vi "Update Controller State.vi"(8 "error in (no error)":errorcluster, 11 "Car Wash Controller Actor in":refnum<class "Car Wash Controller Actor.lvclass">) -> (0 "error out":errorcluster, 3 "Car Wash Controller Actor out":refnum<class "Car Wash Controller Actor.lvclass">)   [LabVIEW 2019, in "Car Wash Controller Actor.lvlib" / "Car Wash Controller Actor.lvclass"]
uses:
  Car Wash Controller Actor.lvclass
  C:/Program Files (x86)/National Instruments/LabVIEW 2019/vi.lib/ActorFramework/Actor/Actor.lvclass
  <vilib>/ActorFramework/Actor/Actor.lvclass/Actor.ctl
  <vilib>/ActorFramework/Message Enqueuer/Message Enqueuer.lvclass/Message Enqueuer.ctl
  Car Wash Controller Actor.lvclass/Car Wash Controller Actor.ctl
  Sim Entry Console Actor/Sim Entry Console Actor/Wash steps selection -Buttons.ctl
  Configuration Database Actor/Configuration Database Actor/DB type.ctl
  Configuration Database Actor/Configuration Database Actor Messages/Select DB Msg/Select DB Msg.lvclass/Select DB Msg.ctl
  Vehicle Position Simulation/Vehicle Position Simulation Messages/Update Vehicle Position Simulation Msg/Update Vehicle Position Simulation Msg.lvclass/Update Vehicle Position Simulation Msg.ctl
  Simulated Wash Display Console Actor/Simulated Wash Display Console Actor Messages/Update Wash Entry Msg/Update Wash Entry Msg.lvclass/Update Wash Entry Msg.ctl
  Simulated Wash Display Console Actor/Simulated Wash Display Console Actor Messages/Update Vehicle Out of Position Msg/Update Vehicle Out of Position Msg.lvclass/Update Vehicle Out of Position Msg.ctl
  Simulated Wash Display Console Actor/Simulated Wash Display Console Actor Messages/Update Car Wash Indicators Msg/Update Car Wash Indicators Msg.lvclass/Update Car Wash Indicators Msg.ctl
  Simulated Wash Display Console Actor/Simulated Wash Display Console Actor Messages/Update Time Remaining Msg/Update Time Remaining Msg.lvclass/Update Time Remaining Msg.ctl
  Sim Entry Console Actor/Simulated Entry Console Actor Messages/Enable Start Msg/Enable Start Msg.lvclass/Enable Start Msg.ctl
  Sim Entry Console Actor/Simulated Entry Console Actor Messages/Enable Wash steps Msg/Enable Wash steps Msg.lvclass/Enable Wash steps Msg.ctl
  State -Enum.ctl
  Car Wash Controller Actor Messages/Set State Msg/Set State Msg.lvclass/Set State Msg.ctl
  <vilib>/ActorFramework/Message Enqueuer/Init from Existing Queue.vi
  <vilib>/ActorFramework/Message Enqueuer/Enqueue.vi
  Configuration Database Actor/Configuration Database Actor Messages/Select DB Msg/Select DB Msg.lvclass
  C:/Program Files (x86)/National Instruments/LabVIEW 2019/vi.lib/ActorFramework/Message/Message.lvclass
  Vehicle Position Simulation/Vehicle Position Simulation Messages/Update Vehicle Position Simulation Msg/Update Vehicle Position Simulation Msg.lvclass
  Simulated Wash Display Console Actor/Simulated Wash Display Console Actor Messages/Update Wash Entry Msg/Update Wash Entry Msg.lvclass
  Simulated Wash Display Console Actor/Simulated Wash Display Console Actor Messages/Update Vehicle Out of Position Msg/Update Vehicle Out of Position Msg.lvclass
  Simulated Wash Display Console Actor/Simulated Wash Display Console Actor Messages/Update Car Wash Indicators Msg/Update Car Wash Indicators Msg.lvclass
  Simulated Wash Display Console Actor/Simulated Wash Display Console Actor Messages/Update Time Remaining Msg/Update Time Remaining Msg.lvclass
  Sim Entry Console Actor/Simulated Entry Console Actor Messages/Enable Start Msg/Enable Start Msg.lvclass
  Sim Entry Console Actor/Simulated Entry Console Actor Messages/Enable Wash steps Msg/Enable Wash steps Msg.lvclass
  Configuration Database Actor/Configuration Database Actor Messages/Read Record Msg/Read Record Msg.lvclass
  Vehicle Position Simulation/Vehicle Position Simulation Messages/Check Vehicle Exit Msg/Check Vehicle Exit Msg.lvclass
  Car Wash Controller Actor Messages/Set State Msg/Set State Msg.lvclass
  <vilib>/ActorFramework/Message Priority Queue/Priority Enqueue.vi
  <vilib>/ActorFramework/Message Enqueuer/Message Enqueuer.lvclass
  <vilib>/ActorFramework/Actor/Actor.lvclass
  Sim Entry Console Actor/Sim Entry Console Actor/Simulated Entry Console Actor.lvclass
  Configuration Database Actor/Configuration Database Actor/Sim Configuration Database Actor.lvclass
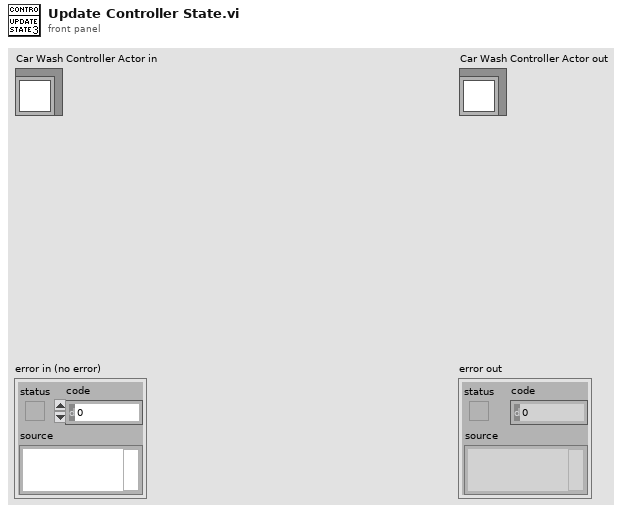
[diagram p1: front panel]
types:
  T1 = typedef "Sim Configuration Database Actor.lvlib/Sim Configuration Database Actor.lvclass/DB type.ctl" = enum16{"Default", "Client"}
  T2 = typedef "Simulated Entry Console Actor.lvlib/Simulated Entry Console Actor.lvclass/Wash steps selection -Buttons.ctl" = cluster{"Under Body Wash":bool, "Bug Remover":bool, "Pre-Soak":bool, "High Pressure Wash (default)":bool, "Low Pressure Wax":bool, "Spot Free Rinse":bool, "Tire Shine Foam":bool, "Air Dry":bool}
  T3 = enum8{"Enabled", "Disabled", "Disabled and Grayed Out"}
  T4 = typedef "Car Wash Controller Actor.lvlib/Car Wash Controller Actor.lvclass/State -Enum.ctl" = enum16{"Initial", "Wait for Start", "Start", "Wait for Vehicle Position", "Wash Step Execution", "Wash Step/Cycle Completion", "Wash Exit", "Wash Abort/Terminate"}
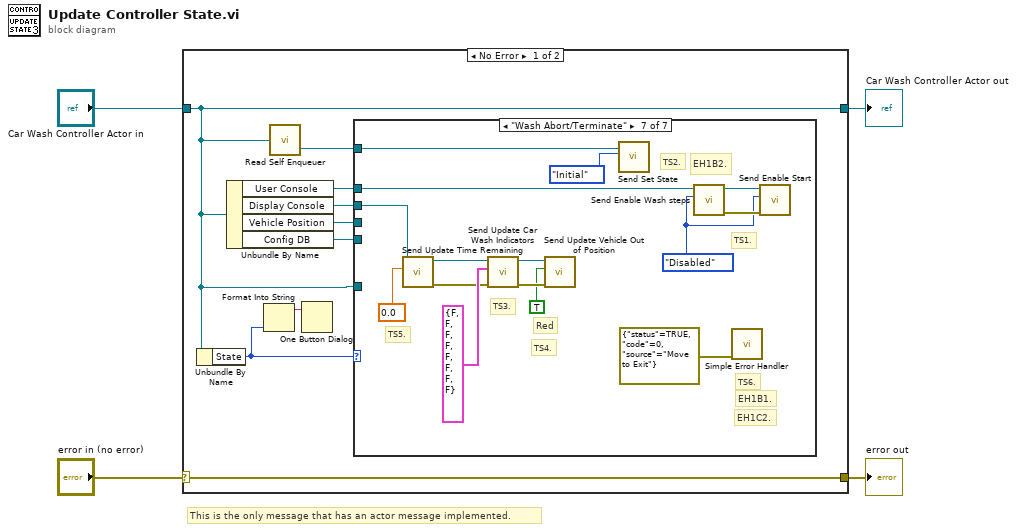
[diagram p0: block diagram]
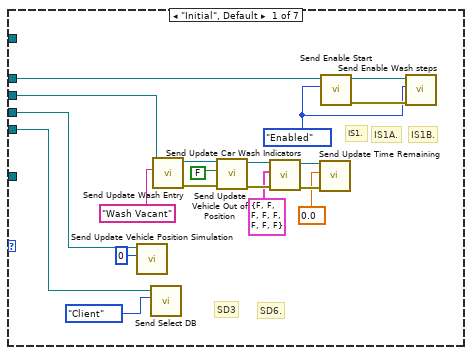
[diagram p2: hidden frame]
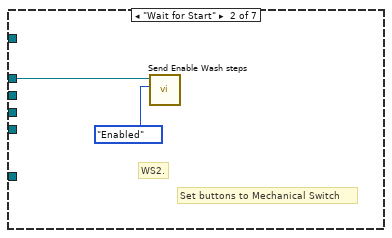
[diagram p3: hidden frame]
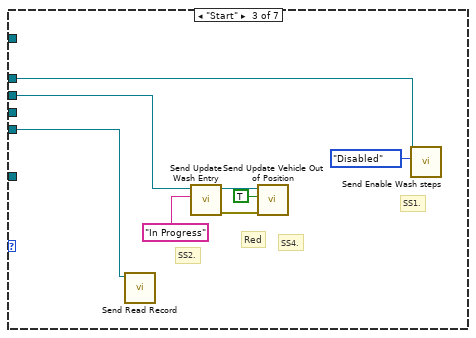
[diagram p4: hidden frame]
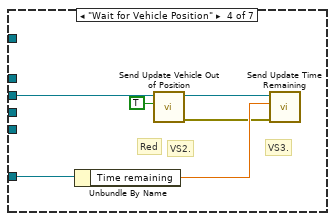
[diagram p5: hidden frame]
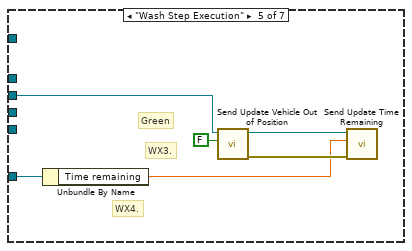
[diagram p6: hidden frame]
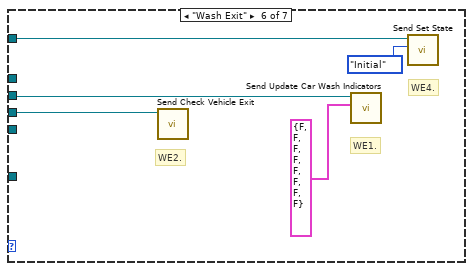
[diagram p7: hidden frame]
diagram:
  # "This is the only message that has an actor message implemented."
  n1 = case shown="No Error" "error in (no error)" {
    selector: "error in (no error)" -> [w13 w76]
    tunnel: [w13 w76] -> w3
    tunnel: [w5 w75] -> w1
    tunnel: "Car Wash Controller Actor in" -> [w5 w75]
    frame No Error {
      n2 = Unbundle By Name(w5) -> ("State"=w7:T4)
      n3 = Unbundle By Name(w5) -> ("User Console"=w11:refnum<class "Message Enqueuer.lvclass">, "Display Console"=w10:refnum<class "Message Enqueuer.lvclass">, "Vehicle Position"=w9:refnum<class "Message Enqueuer.lvclass">, "Config DB"=w8:refnum<class "Message Enqueuer.lvclass">)
      n4 = Format Into String(w7) -> (resulting string=w6:string)  [unwired: 3 in, 1 out]
      n5 = call <vilib>:"Read Self Enqueuer.vi"("Actor"=w5) -> ("Self Enqueuer"=w12:refnum<class "Message Enqueuer.lvclass">)  [unwired: 10 in]
      n6 = One Button Dialog(message=w6) -> ()  [unwired: 1 in, 1 out]
      n7 = case shown="\"Wash Abort/Terminate\"" w7 {
        tunnel: w12 -> [_ _ _ _ _ w57 w61]
        tunnel: w11 -> [w32 w34 w42 _ _ _ w62]
        tunnel: w10 -> [w28 _ w40 w47 w53 w59 w64]
        tunnel: w9 -> [w17 _ _ _ _ w55 _]
        tunnel: w8 -> [w15 _ w35 _ _ _ _]
        tunnel: w5 -> [_ _ _ w45 w50 _ _]
        frame "Initial", Default {
          w29 = T3."Enabled" ("Enabled")
          # "SD6."
          # "SD3"
          # "IS1B."
          # "IS1A."
          # "IS1."
          n8 = call "Send Update Vehicle Position Simulation.vi"("Vehicle Pos"=u32 0, "Message Enqueuer"=w17) -> ()  [unwired: 8 in, 2 out]
          n9 = call "Send Select DB.vi"("DB"=DB_type."Client", "Message Enqueuer"=w15) -> ()  [unwired: 8 in, 2 out]
          n10 = call "Send Update Wash Entry.vi"("Wash Entry"="Wash Vacant", "Message Enqueuer"=w28) -> ("error out"=w25:errorcluster, "Message Enqueuer out"=w26:refnum<class "Message Enqueuer.lvclass">)  [unwired: 8 in]
          n11 = call "Send Update Vehicle Out of Position.vi"("error in (no error)"=w25, "Out of pos?"=FALSE, "Message Enqueuer"=w26) -> ("error out"=w23:errorcluster, "Message Enqueuer out"=w22:refnum<class "Message Enqueuer.lvclass">)  [unwired: 7 in]
          n12 = call "Send Update Car Wash Indicators.vi"("error in (no error)"=w23, "Car Wash Indicators"=T2 {"Under Body Wash"=FALSE, "Bug Remover"=FALSE, "Pre-Soak"=FALSE, "High Pressure Wash (default)"=FALSE, "Low Pressure Wax"=FALSE, "Spot Free Rinse"=FALSE, "Tire Shine Foam"=FALSE, "Air Dry"=FALSE}, "Message Enqueuer"=w22) -> ("error out"=w20:errorcluster, "Message Enqueuer out"=w19:refnum<class "Message Enqueuer.lvclass">)  [unwired: 7 in]
          n13 = call "Send Update Time Remaining.vi"("error in (no error)"=w20, "Timing"=0.0, "Message Enqueuer"=w19) -> ()  [unwired: 7 in, 2 out]
          n14 = call "Send Enable Start.vi"("Enabled"=w29, "Message Enqueuer"=w32) -> ("error out"=w30:errorcluster, "Message Enqueuer out"=w31:refnum<class "Message Enqueuer.lvclass">)  [unwired: 8 in]
          n15 = call "Send Enable Wash steps.vi"("error in (no error)"=w30, "Disabled"=w29, "Message Enqueuer"=w31) -> ()  [unwired: 7 in, 2 out]
        }
        frame "Wait for Start" {
          # "Set buttons to Mechanical Switch"
          # "WS2."
          n16 = call "Send Enable Wash steps.vi"("Disabled"=T3."Enabled", "Message Enqueuer"=w34) -> ()  [unwired: 8 in, 2 out]
        }
        frame "Start" {
          # "SS4."
          # "Red"
          # "SS2."
          # "SS1."
          n17 = call "Send Read Record.vi"("Message Enqueuer"=w35) -> ()  [unwired: 9 in, 2 out]
          n18 = call "Send Update Wash Entry.vi"("Wash Entry"="In Progress", "Message Enqueuer"=w40) -> ("error out"=w36:errorcluster, "Message Enqueuer out"=w38:refnum<class "Message Enqueuer.lvclass">)  [unwired: 8 in]
          n19 = call "Send Update Vehicle Out of Position.vi"("error in (no error)"=w36, "Out of pos?"=TRUE, "Message Enqueuer"=w38) -> ()  [unwired: 7 in, 2 out]
          n20 = call "Send Enable Wash steps.vi"("Disabled"=T3."Disabled", "Message Enqueuer"=w42) -> ()  [unwired: 8 in, 2 out]
        }
        frame "Wait for Vehicle Position" {
          # "VS3."
          # "VS2."
          # "Red"
          n21 = Unbundle By Name(w45) -> ("Time remaining"=w44:dbl)
          n22 = call "Send Update Vehicle Out of Position.vi"("Out of pos?"=TRUE, "Message Enqueuer"=w47) -> ("error out"=w43:errorcluster, "Message Enqueuer out"=w46:refnum<class "Message Enqueuer.lvclass">)  [unwired: 8 in]
          n23 = call "Send Update Time Remaining.vi"("error in (no error)"=w43, "Timing"=w44, "Message Enqueuer"=w46) -> ()  [unwired: 7 in, 2 out]
        }
        frame "Wash Step Execution" {
          # "WX4."
          # "WX3."
          # "Green"
          n24 = Unbundle By Name(w50) -> ("Time remaining"=w49:dbl)
          n25 = call "Send Update Vehicle Out of Position.vi"("Out of pos?"=FALSE, "Message Enqueuer"=w53) -> ("error out"=w51:errorcluster, "Message Enqueuer out"=w52:refnum<class "Message Enqueuer.lvclass">)  [unwired: 8 in]
          n26 = call "Send Update Time Remaining.vi"("error in (no error)"=w51, "Timing"=w49, "Message Enqueuer"=w52) -> ()  [unwired: 7 in, 2 out]
        }
        frame "Wash Exit" {
          # "WE2."
          # "WE4."
          # "WE1."
          n27 = call "Send Check Vehicle Exit.vi"("Message Enqueuer"=w55) -> ()  [unwired: 9 in, 2 out]
          n28 = call "Send Update Car Wash Indicators.vi"("Car Wash Indicators"=T2 {"Under Body Wash"=FALSE, "Bug Remover"=FALSE, "Pre-Soak"=FALSE, "High Pressure Wash (default)"=FALSE, "Low Pressure Wax"=FALSE, "Spot Free Rinse"=FALSE, "Tire Shine Foam"=FALSE, "Air Dry"=FALSE}, "Message Enqueuer"=w59) -> ()  [unwired: 8 in, 2 out]
          n29 = call "Send Set State.vi"("States"=State_-Enum."Initial", "Message Enqueuer"=w57) -> ()  [unwired: 8 in, 2 out]
        }
        frame "Wash Abort/Terminate" {
          w72 = T3."Disabled" ("Disabled")
          # "EH1B2."
          # "EH1C2."
          # "EH1B1."
          # "TS6."
          # "TS5."
          # "TS4."
          # "Red"
          # "TS3."
          # "TS2."
          # "TS1."
          n30 = call "Send Update Time Remaining.vi"("Timing"=0.0, "Message Enqueuer"=w64) -> ("error out"=w66:errorcluster, "Message Enqueuer out"=w67:refnum<class "Message Enqueuer.lvclass">)  [unwired: 8 in]
          n31 = call "Send Update Car Wash Indicators.vi"("error in (no error)"=w66, "Car Wash Indicators"=T2 {"Under Body Wash"=FALSE, "Bug Remover"=FALSE, "Pre-Soak"=FALSE, "High Pressure Wash (default)"=FALSE, "Low Pressure Wax"=FALSE, "Spot Free Rinse"=FALSE, "Tire Shine Foam"=FALSE, "Air Dry"=FALSE}, "Message Enqueuer"=w67) -> ("error out"=w69:errorcluster, "Message Enqueuer out"=w70:refnum<class "Message Enqueuer.lvclass">)  [unwired: 7 in]
          n32 = call "Send Update Vehicle Out of Position.vi"("error in (no error)"=w69, "Out of pos?"=TRUE, "Message Enqueuer"=w70) -> ()  [unwired: 7 in, 2 out]
          n33 = call "Send Set State.vi"("States"=State_-Enum."Initial", "Message Enqueuer"=w61) -> ()  [unwired: 8 in, 2 out]
          n34 = call "Send Enable Wash steps.vi"("Disabled"=w72, "Message Enqueuer"=w62) -> ("error out"=w73:errorcluster, "Message Enqueuer out"=w74:refnum<class "Message Enqueuer.lvclass">)  [unwired: 8 in]
          n35 = call <vilib>:"Simple Error Handler.vi"("error in (no error)"=errorcluster {"status"=TRUE, "code"=0, "source"="Move to Exit"}) -> ()  [unwired: 4 in, 5 out]
          n36 = call "Send Enable Start.vi"("error in (no error)"=w73, "Enabled"=w72, "Message Enqueuer"=w74) -> ()  [unwired: 7 in, 2 out]
        }
      }
    }
    frame Error {
    }
  }
  "error out" <- w3
  "Car Wash Controller Actor out" <- w1
